vi "UniqueLast.vi"   [LabVIEW 2009]
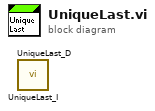
[diagram p0: block diagram]
diagram:
  n1 = call "UniqueLast_I.vi"() -> ()  [unwired: 11 in, 1 out]
  n2 = call "UniqueLast_D.vi"() -> ()  [unwired: 11 in, 1 out]
